vi "AreaInfo.vi"(8 "Error In":errorcluster, 11 "Figure in":refnum<class "Figure.lvclass">) -> (0 "Error Out":errorcluster, 3 "Figure out":refnum<class "Figure.lvclass">)   [LabVIEW 2021, in "Figure.lvclass"]
doc: "Send dialog window with current area of fiugre."
uses:
  Figure.lvclass
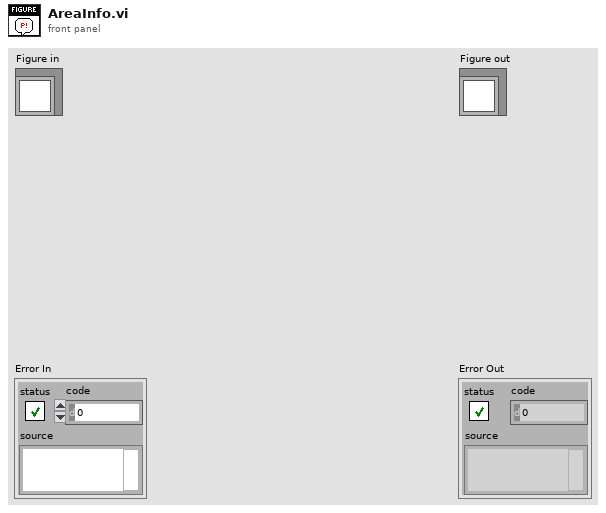
[diagram p1: front panel]
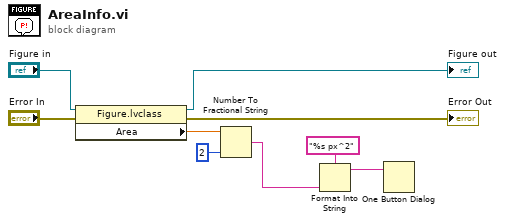
[diagram p0: block diagram]
diagram:
  n1 = property class="Figure.lvclass"(reference="Figure in", error in="Error In") -> (reference out=→"Figure out":refnum<class "Figure.lvclass">, error out=→"Error Out":errorcluster, "Area"=w5:dbl)
  n2 = Number To Fractional String(number=w5, precision (6)=i16 2) -> (F-format string=w2:string)  [unwired: 2 in]
  n3 = Format Into String(format string="%s px^2", w2) -> (resulting string=w1:string)  [unwired: 2 in, 1 out]
  n4 = One Button Dialog(message=w1) -> ()  [unwired: 1 in, 1 out]
